vi "Init Data.vi"(8 "error in (no error)":errorcluster, 10 "Data Object":refnum<class "Factory Plugin Framework.lvclass">, 11 "Servo MSMT in":refnum<class "Servo MSMT.lvclass">) -> (0 "error out":errorcluster, 3 "Servo MSMT out":refnum<class "Servo MSMT.lvclass">)   [LabVIEW 2018, in "Servo MSMT.lvlib" / "Servo MSMT.lvclass"]
uses:
  Servo MSMT.lvclass
  Plugins/FPF.lvlibp/Factory Plugin Framework.lvclass
  Plugins/Measurement Interface.lvlibp/Measurement Interface.lvclass
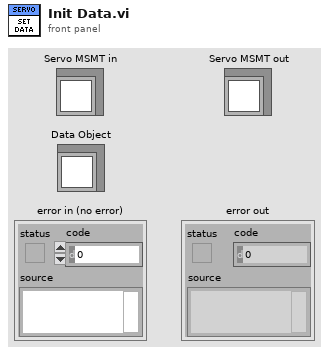
[diagram p1: front panel]
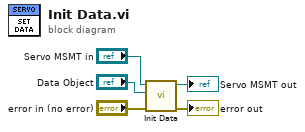
[diagram p0: block diagram]
diagram:
  n1 = call-parent "Init Data.vi"("error in (no error)"="error in (no error)", "Data Object"="Data Object", "Measurement Interface in"="Servo MSMT in") -> ("error out"=→"error out":errorcluster, "Measurement Interface out"=→"Servo MSMT out":refnum<class "Servo MSMT.lvclass">)  [unwired: 7 in]
